vi "WPI_I2CRead.vi"(8 "error in (no error)":errorcluster, 9 "I2CBytesToRead":u8, 10 "I2CRegister":u8[](array[numeric]), 11 "I2CDevRef":T1={"DevStatus"={"status"=FALSE, "code"=0, "source"=""}, "Device Address"=0, "Handle"=0, "I2C Bus"=enum."Invalid"} {"Device Address" format="%.0x"}) -> (0 "error out":errorcluster, 2 "Data Out":u8[](array[numeric]), 3 "I2CDevRef":T1={"DevStatus"={"status"=FALSE, "code"=0, "source"=""}, "Device Address"=0, "Handle"=0, "I2C Bus"=enum."Invalid"} {"Device Address" format="%.0x"})   [LabVIEW 2017]
doc: "Reads between one and four bytes in a single transaction from the I2C sensor you specify.\n\nThis software is licensed. Open the labview\\readme\\WPI Robotics Library Open Source License.txt file for more information."
uses:
  <vilib>/Rock Robotics/WPI/I2C/WPI_I2CDevRef.ctl
  <vilib>/Rock Robotics/SystemInterfaces/i2clib/i2c_bus.ctl
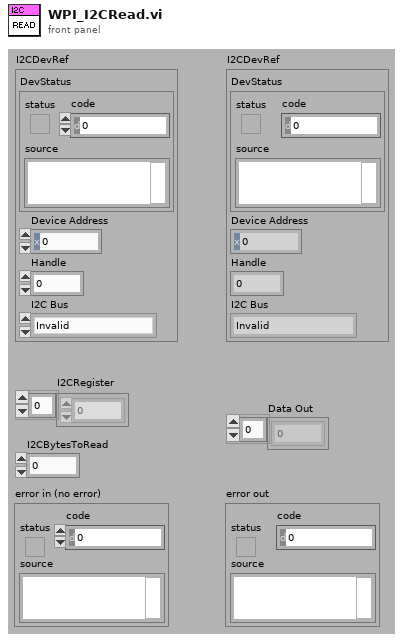
[diagram p1: front panel]
types:
  T1 = typedef "WPI_I2CDevRef.ctl" = cluster{"DevStatus":errorcluster, "Device Address":u8, "Handle":i32, "I2C Bus":T2}
  T2 = typedef "i2c_bus.ctl" = enum16{"I2C On-Board", "I2C MXP", "Invalid"}
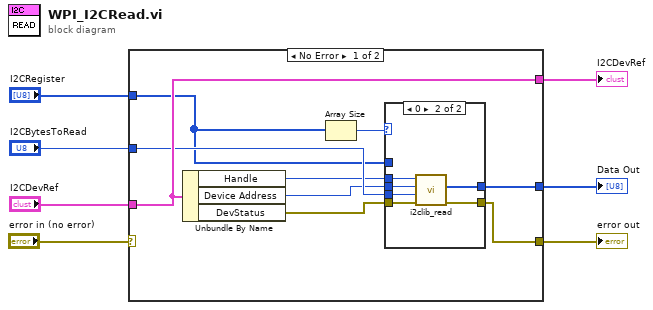
[diagram p0: block diagram]
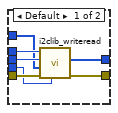
[diagram p2: hidden frame]
diagram:
  n1 = case shown="No Error" "error in (no error)" {
    selector: "error in (no error)" -> [_ w31]
    tunnel: [w9 w31] -> w4
    tunnel: "I2CDevRef" -> [w16 w30]
    tunnel: [w16 w30] -> w1
    tunnel: "I2CBytesToRead" -> [w15 _]
    tunnel: "I2CRegister" -> [w10 _]
    tunnel: [w8 _] -> w2
    frame No Error {
      n2 = Unbundle By Name(w16) -> ("Handle"=w13:i32, "Device Address"=w12:u8, "DevStatus"=w14:errorcluster)
      n3 = Array Size(array=w10) -> (size(s)=w11:i32)
      n4 = case shown="0" w11 {
        tunnel: w15 -> [w19 w29]
        tunnel: w14 -> [w20 w28]
        tunnel: w13 -> [w23 w27]
        tunnel: w12 -> [w22 w26]
        tunnel: w10 -> [w21 _]
        tunnel: [w18 w25] -> w8
        tunnel: [w17 w24] -> w9
        frame Default {
          n5 = call <vilib>:"i2clib_writeread.vi"("recv_size"=w19, "error in (no error)"=w20, "send_data"=w21, "dev_addr"=w22, "I2C Reference"=w23) -> ("error out"=w17:errorcluster, "recv_data"=w18:u8[])  [unwired: 4 in, 1 out]
        }
        frame 0 {
          n6 = call <vilib>:"i2clib_read.vi"("error in (no error)"=w28, "recv_size"=w29, "dev_addr"=w26, "I2C Reference"=w27) -> ("error out"=w24:errorcluster, "recv_data"=w25:u8[])  [unwired: 5 in, 1 out]
        }
      }
    }
    frame Error {
    }
  }
  "error out" <- w4
  "Data Out" <- w2
  "I2CDevRef" <- w1
